vi "CallRelativeVI.vi"(2 "error in (no error)":errorcluster, 3 "VI Path":path) -> (0 "error out":errorcluster)   [LabVIEW 2014]
uses:
  globals/AzCamGlobals.vi
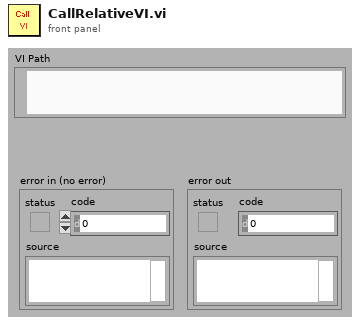
[diagram p1: front panel]
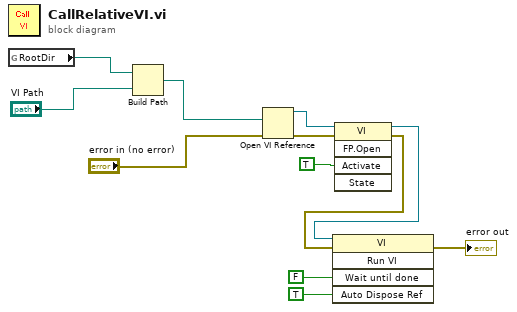
[diagram p0: block diagram]
diagram:
  n1 = global read "AzCamGlobals.vi" "RootDir"() -> (w3:path)
  n2 = Build Path(base path=w3, name or relative path="VI Path") -> (appended path=w4:path)
  n3 = Open VI Reference(vi path=w4, error in (no error)="error in (no error)") -> (vi reference=w7:refnum<vi>, error out=w10:errorcluster)  [unwired: 4 in]
  n4 = invoke class="VI" method="FP.Open"(reference=w7, error in=w10, "Activate"=TRUE ("Activate?")) -> (reference out=w9:refnum<vi>, error out=w8:errorcluster)  [unwired: 2 in, 3 out]
  n5 = invoke class="VI" method="Run VI"(reference=w9, error in=w8, "Wait until done"=FALSE, "Auto Dispose Ref"=TRUE) -> (error out=→"error out":errorcluster)  [unwired: 1 in, 4 out]
